vi "Get Class Name.vi"(8 "error in (no error)":errorcluster, 11 "Search Result in":refnum<class "Search Result.lvclass">) -> (0 "error out":errorcluster, 2 "Class Name":string, 3 "Search Result out":refnum<class "Search Result.lvclass">)   [LabVIEW 2016, in "Better Search.lvlib" / "Search Result.lvclass"]
uses:
  Search Result.lvclass
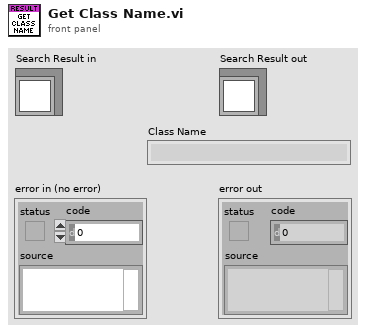
[diagram p1: front panel]
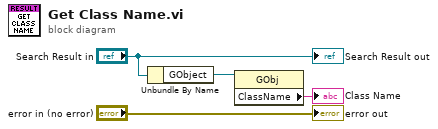
[diagram p0: block diagram]
diagram:
  n1 = Unbundle By Name("Search Result in") -> ("GObject"=w2:refnum<vi>)
  n2 = property class="GObj"(reference=w2) -> ("ClassName"=→"Class Name":string)  [unwired: 1 in, 2 out]
  "error out" <- "error in (no error)"
  "Search Result out" <- "Search Result in"
